vi "Collection.vi"(8 "error in (no error)":errorcluster, 10 "Array":refnum<class "Readable.lvclass">[](array[class]), 11 "Collection.lvclass in":refnum<class "Collection.lvclass">) -> (0 "error out":errorcluster, 3 "Collection.lvclass out":refnum<class "Collection.lvclass">)   [LabVIEW 2009, in "Collection.lvclass"]
uses:
  Collection.lvclass
  Readable/Readable.lvclass
  Readable/Channel Units.ctl
  Collection.lvclass/Collection.ctl
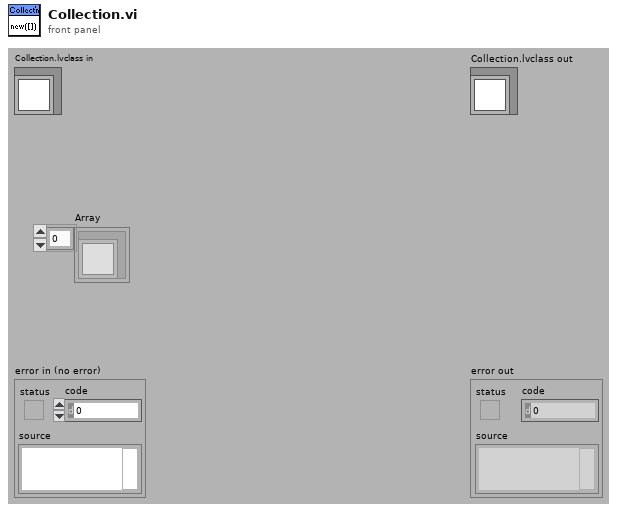
[diagram p1: front panel]
types:
  T1 = typedef "Readable.lvclass/Channel Units.ctl" = string[]
  T2 = typedef "Readable.lvclass/Channel Names.ctl" = string[]
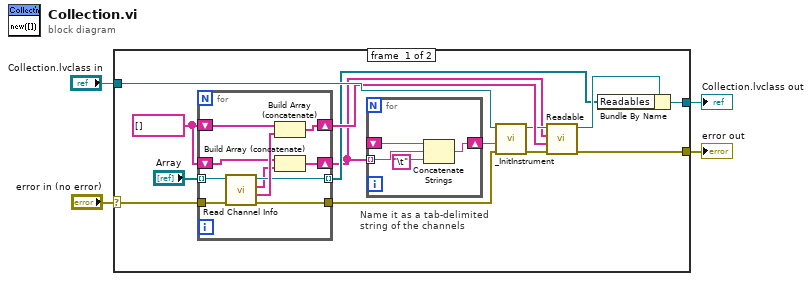
[diagram p0: block diagram]
diagram:
  n1 = case shown="No Error" "error in (no error)" {
    selector: "error in (no error)" -> [w12 w33]
    tunnel: [w11 w33] -> w3
    tunnel: [w18 w34] -> w1
    tunnel: "Collection.lvclass in" -> [w17 w34]
    frame #0 {
      w13 = T1 [] ("Channel Units")
      n2 = for {
        tunnel: "Array" -> [w32] mode=indexing
        shift-right: [w31] -> w14
        shift-left: w13 -> [w29]
        shift-right: [w28] -> w8
        shift-left: w13 -> [w26]
        tunnel: [w27] -> w10 mode=indexing
        tunnel: w12 -> [w25]
        tunnel: [w24] -> w5
        n3 = call "Read Channel Info.vi"("error in (no error)"=w25, "Readable.lvclass in"=w32) -> ("error out"=w24:errorcluster, "Channel Units"=w30:T1, "Channel Names"=w23:T2, "Readable.lvclass out"=w27:refnum<class "Readable.lvclass">)  [unwired: 5 in, 1 out]
        n4 = Build Array (concatenate)(w29, w30) -> (w31:T1)
        n5 = Build Array (concatenate)(w26, w23) -> (w28:T2)
      }
      n6 = for "Name it as a tab-delimited\nstring of the channels" {
        shift-right: [w21] -> w7
        shift-left: _ -> [w22]
        tunnel: w8 -> [w19] mode=indexing
        n7 = Concatenate Strings(w22, w19, "\t") -> (w21:string)
      }
      n8 = call-dynamic "_InitInstrument.vi"("error in (no error)"=w5, "Name"=w7, "Instrument in"=w17) -> ("error out"=w6:errorcluster, "Instrument out"=w9:refnum<class "Collection.lvclass">)  [unwired: 7 in]
      n9 = call "Readable.vi"("error in (no error)"=w6, "Channel Units"=w14, "Channel Names"=w8, "Readable in"=w9) -> ("error out"=w11:errorcluster, "Readable out"=w16:refnum<class "Collection.lvclass">)  [unwired: 6 in]
      n10 = Bundle By Name(cluster=w16, "Readables"=w10) -> (w18:refnum<class "Collection.lvclass">)
    }
    frame #1 {
    }
  }
  "error out" <- w3
  "Collection.lvclass out" <- w1
